vi "Handle SmartMotor ASCII strings.vi"(3 "error in (no error)":errorcluster, 5 "String in":string) -> (0 "error out":errorcluster, 2 "String out":string)   [LabVIEW 2017]
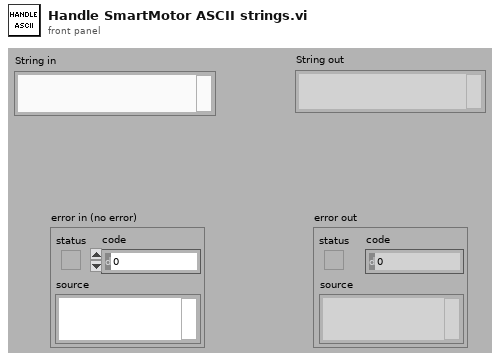
[diagram p1: front panel]
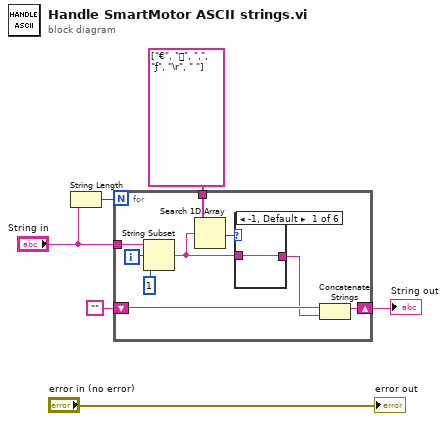
[diagram p0: block diagram]
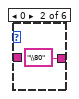
[diagram p2: hidden frame]
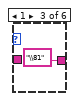
[diagram p3: hidden frame]
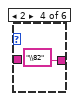
[diagram p4: hidden frame]
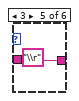
[diagram p5: hidden frame]
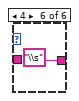
[diagram p6: hidden frame]
diagram:
  n1 = String Length(string="String in") -> (length=w5:i32)
  n2 = for {
    N: w5 -> [_]
    shift-right: [w14] -> w1
    shift-left: "" -> [w13]
    tunnel: "String in" -> [w12]
    tunnel: string[] ["€", "", "‚", "ƒ", "\r", " "] -> [w10]
    i -> [w11]
    n3 = String Subset(string=w12, offset (0)=w11, length (rest)=1 ("length (rest)")) -> (substring=w8:string)
    n4 = Search 1D Array(1D array=w10, element=w8) -> (index of element=w9:i32)  [unwired: 1 in]
    n5 = case shown="-1, Default" w9 {
      tunnel: w8 -> [w16 _ _ _ _ _]
      tunnel: [w16 "\\80" "\\81" "\\82" "\\r" "\\s"] -> w7
      frame -1, Default {
      }
      frame 0 {
      }
      frame 1 {
      }
      frame 2 {
      }
      frame 3 {
      }
      frame 4 {
      }
    }
    n6 = Concatenate Strings(w13, w7) -> (w14:string)
  }
  "String out" <- w1
  "error out" <- "error in (no error)"
